vi "Read Load Path.vi"(8 "error in (no error)":errorcluster, 11 "EST Output in":refnum<class "EST Output.lvclass">) -> (0 "error out":errorcluster, 2 "Load Path":path, 3 "EST Output out":refnum<class "EST Output.lvclass">)   [LabVIEW 2015, in "EST Output.lvclass"]
uses:
  EST Output.lvclass
  EST Output.lvclass/EST Output.ctl
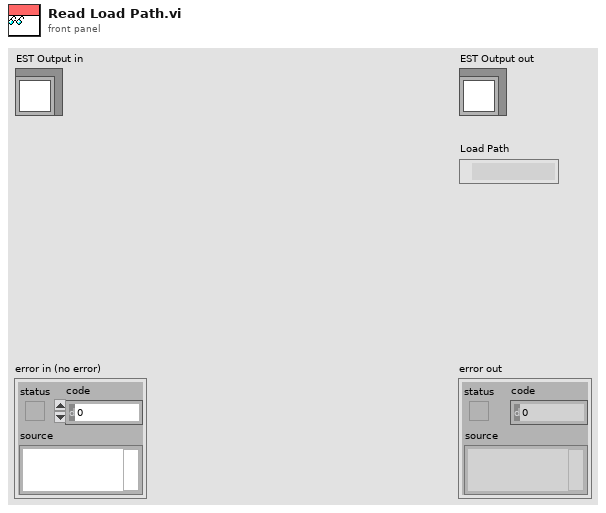
[diagram p1: front panel]
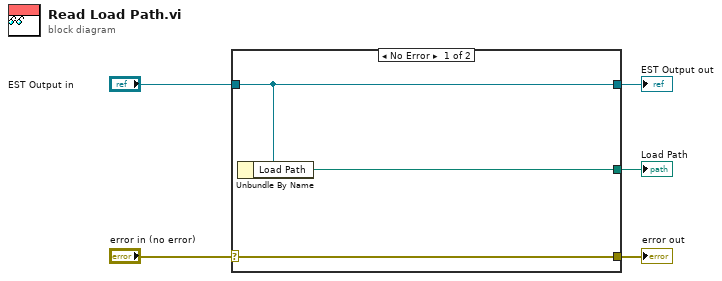
[diagram p0: block diagram]
diagram:
  n1 = case shown="No Error" "error in (no error)" {
    selector: "error in (no error)" -> [w8 w9]
    tunnel: [w8 w9] -> w4
    tunnel: [w7 w10] -> w2
    tunnel: "EST Output in" -> [w7 w10]
    tunnel: [w6 _] -> w1
    frame No Error {
      n2 = Unbundle By Name(w7) -> ("Load Path"=w6:path)
    }
    frame Error {
    }
  }
  "error out" <- w4
  "EST Output out" <- w2
  "Load Path" <- w1
